vi "Panel-RasterAO.vi"() -> ()   [LabVIEW 2009]
uses:
  Instruments/RTC/Api/TelemetryServer/TelemetryServer_Global.vi
panel:
  in  "Tab Control":enum32{"Main", "Debug"}(tab)
  out "Sum":dbl[][](graph)
  out "FWHM Y (m\")":dbl format="%#.0f"
  out "FWHM X (m\")":dbl format="%#.0f"
  out "Y (m\")":dbl format="%#.0f"
  out "X (m\")":dbl format="%#.0f"
  out "Up":dbl[][](graph)
  out "Down":dbl[][](graph)
  out "Difference":dbl[][](graph)
  out "Pixel rate":dbl
  in  "Time Shift":dbl=-0.01
  in  "AO":enum16{"K1", "K2"}(ring)
  in  "Amp (m\")":dbl=200.0
  in  "Freq":dbl=1.0 format="%.3g"
  in  "N":i32=5
  in  "stop":bool
  # "+Y"
  # "+X"
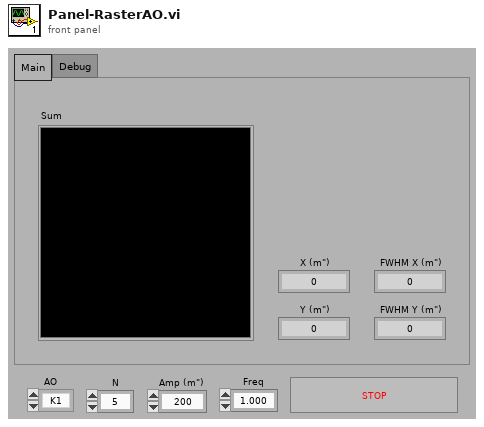
[diagram p1: front panel]
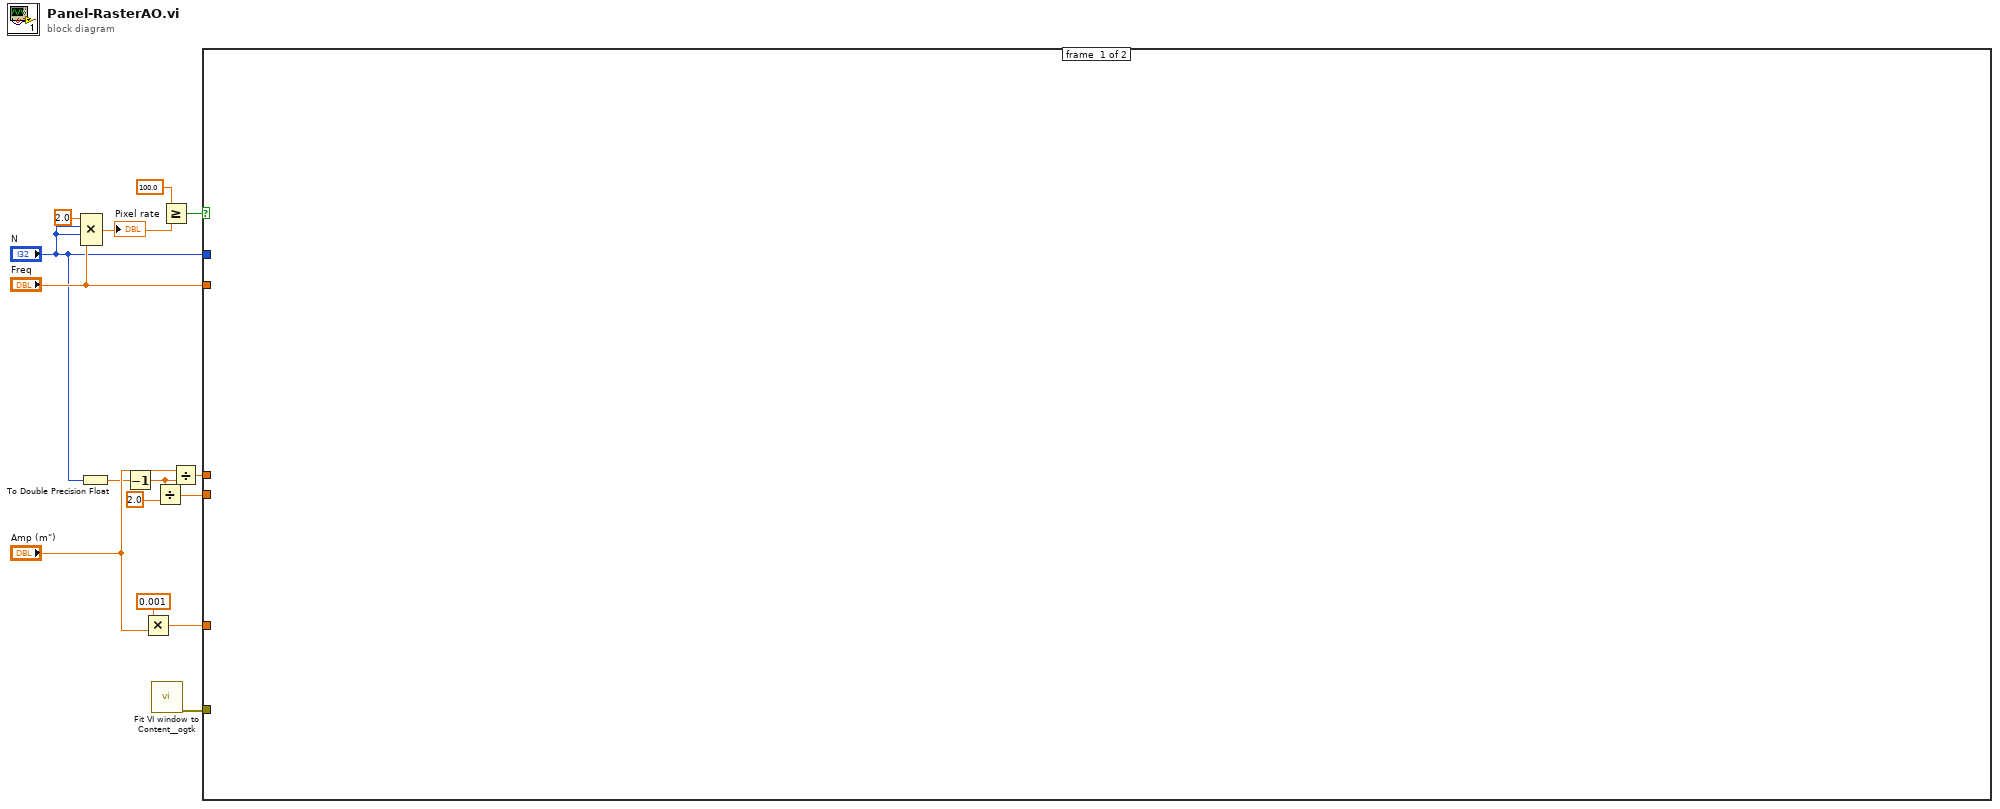
[diagram p0: block diagram]
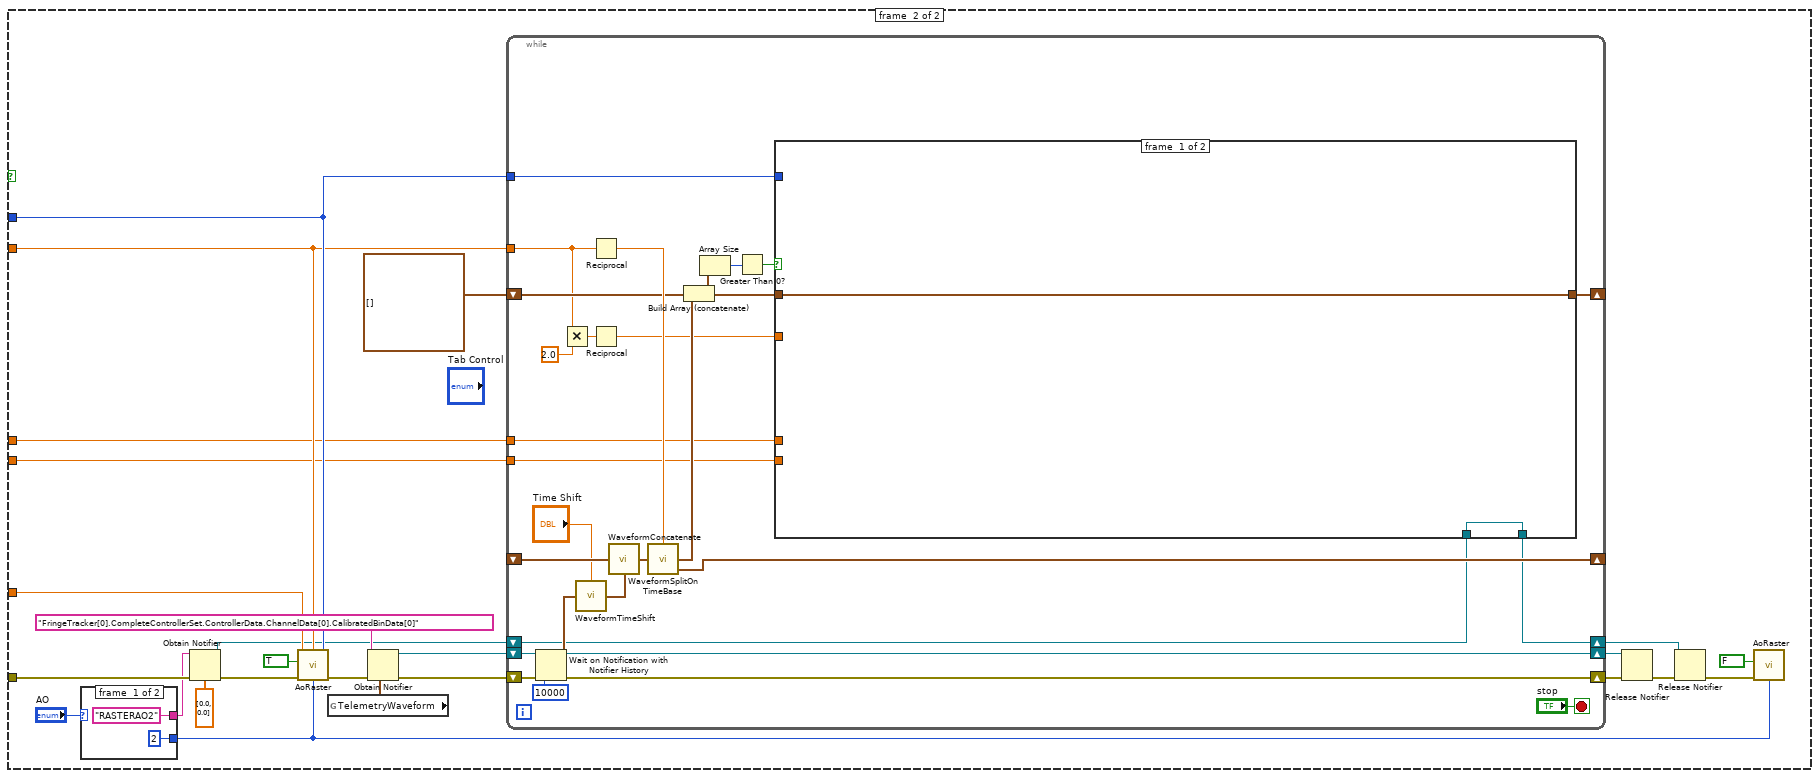
[diagram p2: hidden frame]
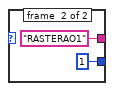
[diagram p3: hidden frame]
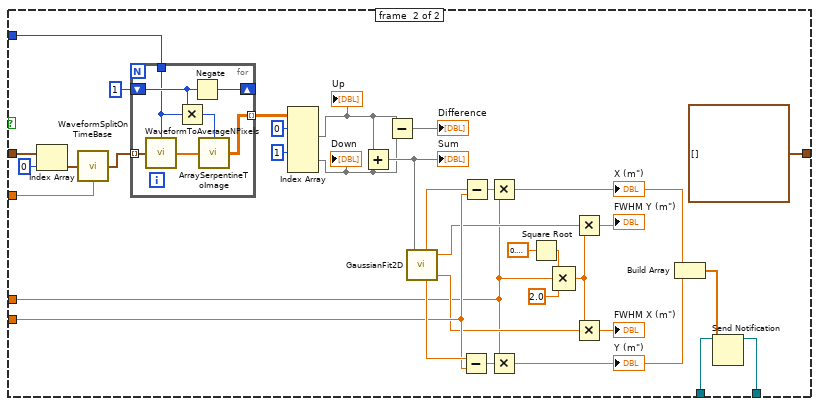
[diagram p4: hidden frame]
diagram:
  n1 = Compound Arithmetic op=MULTIPLY(2.0 ("value"), "N", "N", "Freq") -> (w11:dbl)
  "Pixel rate" <- w11
  n2 = To Double Precision Float(number="N") -> (double precision float=w2:dbl)
  n3 = Decrement(x=w2) -> (x-1=w6:dbl)
  n4 = Multiply(x=0.001, y="Amp (m\")") -> (x*y=w4:dbl)
  n5 = call <userlib>:"Fit VI window to Content__ogtk.vi"() -> ("error out"=w1:errorcluster)  [unwired: 3 in, 4 out]
  n6 = Divide(x=w6, y=2.0) -> (x/y=w5:dbl)
  n7 = Greater Or Equal?(x=100.0, y=w11) -> (x >= y?=w12:bool)
  n8 = Divide(x="Amp (m\")", y=w6) -> (x/y=w9:dbl)
  n9 = case shown="True" w12 {
    tunnel: w4 -> [_ w33]
    tunnel: "N" -> [_ w30]
    tunnel: "Freq" -> [_ w29]
    tunnel: w9 -> [_ w27]
    tunnel: w5 -> [_ w26]
    tunnel: w1 -> [_ w25]
    frame #0 {
    }
    frame #1 {
      n10 = case shown="\"K1\"" "AO" {
        tunnel: ["RASTERAO2" "RASTERAO1"] -> w23
        tunnel: [2 1] -> w16
        frame #0 {
        }
        frame #1 {
        }
      }
      n11 = Obtain Notifier(name (unnamed)=w23, notification data type=dbl[] [0.0, 0.0], error in (no error)=w25) -> (notifier out=w21:refnum<notifier>, error out=w24:errorcluster)  [unwired: 1 in, 1 out]
      n12 = call "AoRaster.vi"("N"=w30, "Frequency"=w29, "Amplitude"=w33, "On / Off"=TRUE, "AO Index"=w16, "error in (no error)"=w24) -> ("error out"=w34:errorcluster)  [unwired: 2 in, 1 out]
      n13 = global read "TelemetryServer_Global.vi" "TelemetryWaveform"() -> (w40:waveform(dbl))
      n14 = Obtain Notifier(name (unnamed)="FringeTracker[0].CompleteControllerSet.ControllerData.ChannelData[0].CalibratedBinData[0]" ("Telemetry"), notification data type=w40, error in (no error)=w34) -> (notifier out=w38:refnum<notifier>, error out=w37:errorcluster)  [unwired: 1 in, 1 out]
      n15 = while {
        shift-right: [w68] -> w35
        shift-left: w37 -> [w71]
        shift-right: [w69] -> w36
        shift-left: w38 -> [w72]
        shift-right: [w65] -> _
        shift-left: _ -> [w66]
        tunnel: w30 -> [w59]
        tunnel: w29 -> [w46]
        shift-right: [w58] -> _
        shift-left: waveform(dbl)[] [] -> [w57]
        tunnel: w27 -> [w53]
        tunnel: w26 -> [w52]
        shift-right: [w50] -> w18
        shift-left: w21 -> [w51]
        stop <- "stop" stop-if-true
        n16 = Wait on Notification with Notifier History(0:w72, 2:10000 ("timeout in ms (-1)"), 3:w71) -> (8:w69:refnum<notifier>, 9:w62:waveform(dbl), 11:w68:errorcluster)  [unwired: 2 out]
        n17 = Multiply(x=w46, y=2.0) -> (x*y=w47:dbl)
        n18 = call "WaveformTimeShift.vi"("Waveform In"=w62, "Time Shift"="Time Shift") -> ("Waveform Out"=w61:waveform(dbl))
        n19 = Reciprocal(x=w46) -> (1/x=w63:dbl)
        n20 = Reciprocal(x=w47) -> (1/x=w45:dbl)
        n21 = call "WaveformConcatenate.vi"("Before"=w66, "After"=w61) -> ("Before After"=w60:waveform(dbl))
        n22 = call "WaveformSplitOnTimeBase.vi"("Waveform In"=w60, "dt"=w63) -> ("Waveform Array"=w56:waveform(dbl)[], "Residual After"=w65:waveform(dbl))  [unwired: 1 out]
        n23 = Build Array (concatenate)(w57, w56) -> (w55:waveform(dbl)[])
        n24 = Array Size(array=w55) -> (size(s)=w48:i32)
        n25 = Greater Than 0?(x=w48) -> (x > 0?=w54:bool)
        n26 = case shown="True" w54 {
          tunnel: w59 -> [_ w104]
          tunnel: w55 -> [w74 w103]
          tunnel: [w74 waveform(dbl)[] []] -> w58
          tunnel: w53 -> [_ w84]
          tunnel: w52 -> [_ w94]
          tunnel: w51 -> [w73 w83]
          tunnel: [w73 w79] -> w50
          tunnel: w45 -> [_ w77]
          frame #0 {
          }
          frame #1 {
            n27 = Index Array(array=w103, index=0) -> (element=w76:waveform(dbl))
            n28 = call "WaveformSplitOnTimeBase.vi"("Waveform In"=w76, "dt"=w77) -> ("Waveform Array"=w75:waveform(dbl)[])  [unwired: 2 out]
            n29 = for {
              tunnel: [w114] -> w105 mode=indexing
              tunnel: w104 -> [w113]
              tunnel: w75 -> [w110] mode=indexing
              shift-right: [w109] -> _
              shift-left: 1 -> [w115]
              n30 = call "WaveformToAverageNPixels.vi"("Waveform"=w110, "N"=w113) -> ("Pixels"=w112:dbl[])
              n31 = Multiply(x=w115, y=w113) -> (x*y=w111:i32)
              n32 = Negate(x=w115) -> (-x=w109:i32)
              n33 = call "ArraySerpentineToImage.vi"("DataIn"=w112, "N"=w111) -> ("DataOut"=w114:dbl[][])
            }
            n34 = Index Array(array=w105, index (dim 0) #1=0 ("index (row)"), index (dim 0) #2=1 ("index (row)")) -> (element #1=w97:dbl[][], element #2=w98:dbl[][])  [unwired: 4 in]
            "Down" <- w98
            "Up" <- w97
            n35 = Add(x=w97, y=w98) -> (x+y=w99:dbl[][])
            "Sum" <- w99
            n36 = Subtract(x=w97, y=w98) -> (x-y=→"Difference":dbl[][])
            n37 = call "GaussianFit2D.vi"("Image"=w99) -> ("b"=w85:dbl, "y"=w95:dbl, "a"=w86:dbl, "x"=w96:dbl)  [unwired: 2 out]
            n38 = Subtract(x=w95, y=w94) -> (x-y=w92:dbl)
            n39 = Subtract(x=w96, y=w94) -> (x-y=w93:dbl)
            n40 = Multiply(x=w93, y=w84) -> (x*y=w82:dbl)
            "X (m\")" <- w82
            n41 = Multiply(x=w92, y=w84) -> (x*y=w81:dbl)
            "Y (m\")" <- w81
            n42 = Square Root(x=0.6931471805599453) -> (sqrt(x)=w88:dbl)
            n43 = Compound Arithmetic op=MULTIPLY(w88, w84, 2.0 ("y")) -> (w89:dbl)
            n44 = Multiply(x=w86, y=w89) -> (x*y=→"FWHM Y (m\")":dbl)
            n45 = Multiply(x=w85, y=w89) -> (x*y=→"FWHM X (m\")":dbl)
            n46 = Build Array(w82, w81) -> (w80:dbl[])
            n47 = Send Notification(notification=w80, notifier=w83) -> (notifier out=w79:refnum<notifier>)  [unwired: 1 in, 1 out]
          }
        }
      }
      n48 = Release Notifier(notifier=w36, error in (no error)=w35) -> (error out=w20:errorcluster)  [unwired: 3 out]
      n49 = Release Notifier(notifier=w18, error in (no error)=w20) -> (error out=w19:errorcluster)  [unwired: 3 out]
      n50 = call "AoRaster.vi"("On / Off"=FALSE, "AO Index"=w16, "error in (no error)"=w19) -> ()  [unwired: 5 in, 2 out]
    }
  }
